vi "UDPtrigger.vi"(9 "occurrence":refnum<k4>, 10 "UDP_port":u16=53000) -> (0 "packet_latency_ms":dbl format="%#.10g", 1 "time_when_received_sec":dbl format="%#.10f", 2 "packet_timestamp_sec":dbl format="%#.10g", 3 "Trigger":bool, 4 "error out":errorcluster)   [LabVIEW 2019]
panel:
  out "UDP_packet_contents":string="0"
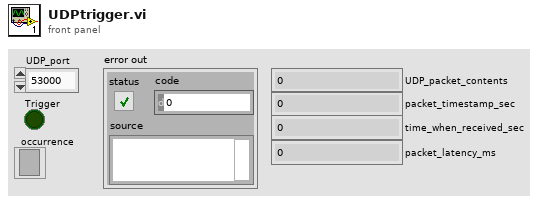
[diagram p1: front panel]
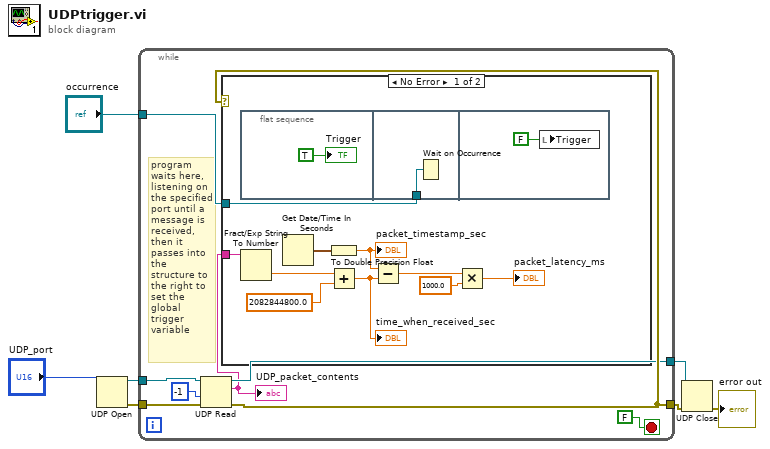
[diagram p0: block diagram]
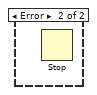
[diagram p2: hidden frame]
diagram:
  n1 = UDP Open(11:"UDP_port") -> (port=w3:refnum<k16>, 0:w4:errorcluster)  [unwired: 4 in, 1 out]
  n2 = while {
    tunnel: [w15] -> w7
    tunnel: [w14] -> w6
    tunnel: w4 -> [w13]
    tunnel: w3 -> [w12]
    tunnel: "occurrence" -> [w8]
    stop <- FALSE stop-if-true
    # "program waits here, listening on the specified port until a message is received, then it passes into the structure to the right to set the global trigger variable"
    n3 = UDP Read(connection ID=w12, timeout ms (25000)=-1, 8:w13) -> (data out=w10:string, error out=w15:errorcluster, 3:w14:refnum<k16>)  [unwired: 1 in, 2 out]
    "UDP_packet_contents" <- w10
    n4 = case shown="No Error" w15 {
      tunnel: w10 -> [w25 _]
      tunnel: w8 -> [w16 _]
      frame No Error {
        n5 = flat-sequence {
          tunnel: w16 -> [w27]
          frame #0 {
            "Trigger" <- TRUE
          }
          frame #1 {
            n6 = Wait on Occurrence(2:w27) -> ()  [unwired: 2 in, 1 out]
          }
          frame #2 {
            n7 = local write "Trigger"(FALSE) -> ()
          }
        }
        n8 = Fract/Exp String To Number(string=w25) -> (number=w19:dbl)  [unwired: 3 in, 1 out]
        n9 = Get Date/Time In Seconds() -> (seconds since 1Jan1904=w23:timestamp)
        n10 = To Double Precision Float(number=w23) -> (double precision float=w17:dbl)
        "packet_timestamp_sec" <- w17
        n11 = Add(x=w19, y=2082844800.0) -> (x+y=w18:dbl)
        "time_when_received_sec" <- w18
        n12 = Subtract(x=w17, y=w18) -> (x-y=w24:dbl)
        n13 = Multiply(x=w24, y=1000.0) -> (x*y=→"packet_latency_ms":dbl)
      }
      frame Error {
        n14 = Stop() -> ()  [unwired: 1 in]
      }
    }
  }
  n15 = UDP Close(connection ID=w6, 8:w7) -> (error out=→"error out":errorcluster)  [unwired: 1 out]
